vi "Save.vi"(6 "SetDif(MPa)":dbl, 9 "SetPressure(MPa)":dbl, 10 "SafePre":dbl, 11 "SetVol":dbl) -> (2 "error out":errorcluster caption="错误输出", 3 "refnum out":T1 caption="引用句柄输出")   [LabVIEW 2014]
uses:
  <vilib>/Utility/config.llb/Config Data RefNum.ctl
  <vilib>/Utility/config.llb/Write Key (Double).vi
  <vilib>/Utility/config.llb/NI_LVConfig.lvlib
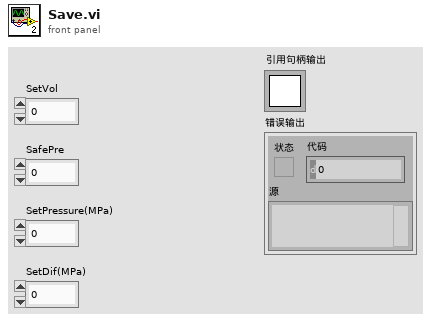
[diagram p1: front panel]
types:
  T1 = typedef "NI_LVConfig.lvlib/Config Data RefNum.ctl" = refnum<k1>
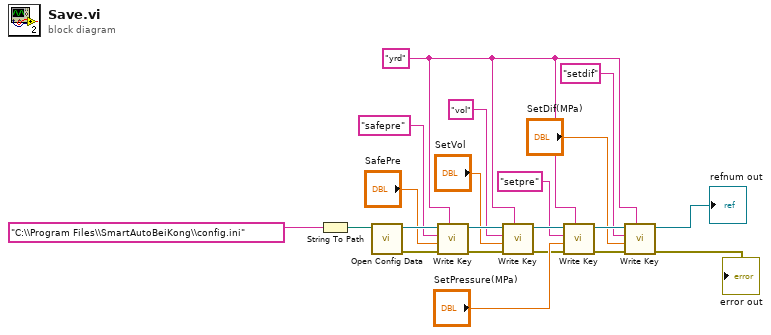
[diagram p0: block diagram]
diagram:
  w7 = "yrd" ("section")
  n1 = String To Path(string="C:\\Program Files\\SmartAutoBeiKong\\config.ini") -> (path=w20:path)
  n2 = call <vilib>:"Open Config Data.vi"("configuration file path"=w20) -> ("error out"=w13:errorcluster, "refnum"=w19:T1)  [unwired: 2 in, 7 out]
  n3 = call-poly <vilib>:"Write Key.vi"("section"=w7, "error in (no error)"=w13, "value"="SafePre", "key"="safepre", "refnum"=w19) -> ("error out"=w12:errorcluster, "refnum out"=w16:T1)  [unwired: 4 in, 1 out]
  n4 = call-poly <vilib>:"Write Key.vi"("section"=w7, "error in (no error)"=w12, "value"="SetVol", "key"="vol", "refnum"=w16) -> ("error out"=w4:errorcluster, "refnum out"=w11:T1)  [unwired: 4 in, 1 out]
  n5 = call-poly <vilib>:"Write Key.vi"("section"=w7, "error in (no error)"=w4, "value"="SetPressure(MPa)", "key"="setpre", "refnum"=w11) -> ("error out"=w3:errorcluster, "refnum out"=w8:T1)  [unwired: 4 in, 1 out]
  n6 = call-poly <vilib>:"Write Key.vi"("section"=w7, "error in (no error)"=w3, "value"="SetDif(MPa)", "key"="setdif", "refnum"=w8) -> ("error out"=→"error out":errorcluster, "refnum out"=→"refnum out":T1)  [unwired: 4 in, 1 out]
